vi "Write Curve.vi"(6 "LinkData":T2, 8 "Error In":errorcluster, 9 "Characteristic Curve Values":dbl[](array[numeric]), 10 "Link":T3, 11 "WorkspaceManager":T1) -> (0 "Error Out":errorcluster, 3 "WorkspaceManager out":T1)   [LabVIEW 2011]
uses:
  Controls/ECUMC Item.ctl
  Controls/LinkData.ctl
  <vilib>/NI Veristand/Execution/Workspace/WorkspaceAPI.ctl
  NationalInstruments.VeriStand.ClientAPI
  <vilib>/ECUMC/NIVS/Support Files.llb/Set Char Data (1d, TCP).vi
  <vilib>/NI Veristand/Execution/Workspace/NI VeriStand - Set Multiple Channel Values.vi
  <vilib>/NI Veristand/Execution/Workspace/NI_VS Workspace ExecutionAPI.lvlib
  <vilib>/ECUMC/NIVS/XCPCCP Add-On Execution API.lvlib
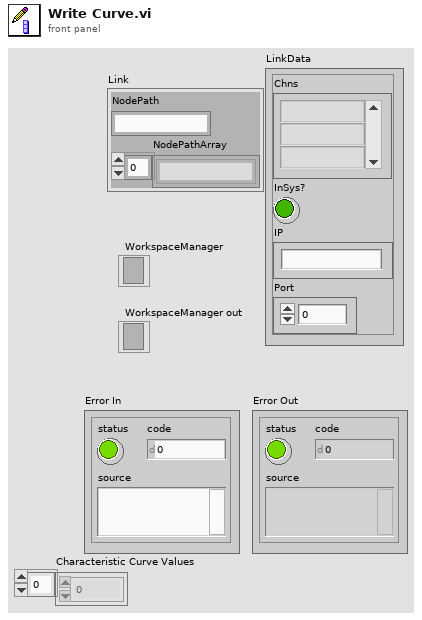
[diagram p1: front panel]
types:
  T1 = typedef "NI_VS Workspace ExecutionAPI.lvlib/WorkspaceAPI.ctl" = refnum<k24>
  T2 = typedef "LinkData.ctl" = cluster{"Chns":string[], "InSys?":bool, "IP":string, "Port":u16}
  T3 = typedef "ECUMC Item.ctl" = cluster{"NodePath":string, "NodePathArray":string[]}
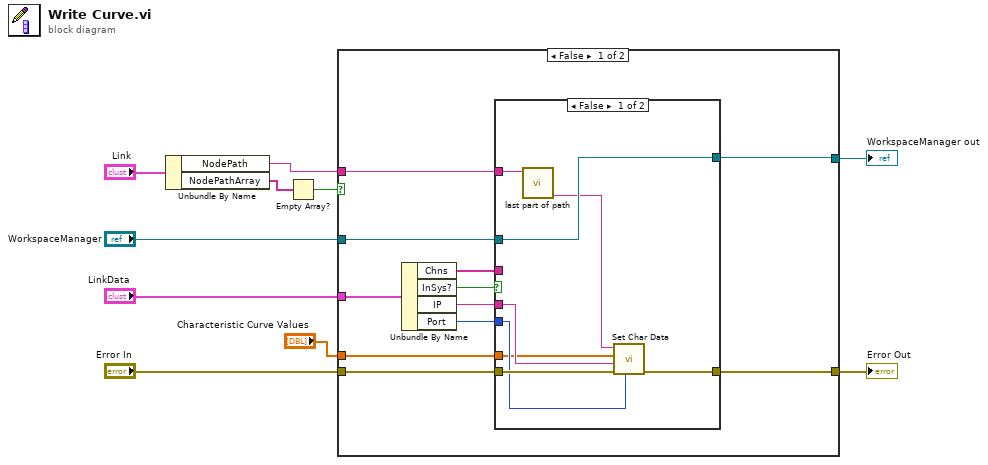
[diagram p0: block diagram]
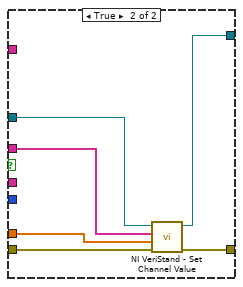
[diagram p2: hidden frame]
diagram:
  n1 = Unbundle By Name("Link") -> ("NodePath"=w7:string, "NodePathArray"=w4:string[])
  n2 = Empty Array?(array=w4) -> (empty?=w3:bool)
  n3 = case shown="False" w3 {
    tunnel: "LinkData" -> [w21 _]
    tunnel: "Error In" -> [w18 w37]
    tunnel: w7 -> [w11 _]
    tunnel: "WorkspaceManager" -> [w15 w36]
    tunnel: [w14 w37] -> w5
    tunnel: [w13 w36] -> w2
    tunnel: "Characteristic Curve Values" -> [w12 _]
    frame False {
      n4 = Unbundle By Name(w21) -> ("Chns"=w19:string[], "InSys?"=w20:bool, "IP"=w17:string, "Port"=w16:u16)
      n5 = case shown="False" w20 {
        tunnel: w19 -> [_ w31]
        tunnel: w15 -> [w25 w35]
        tunnel: w18 -> [w29 w34]
        tunnel: [w28 w33] -> w14
        tunnel: w17 -> [w27 _]
        tunnel: w16 -> [w26 _]
        tunnel: [w25 w32] -> w13
        tunnel: w12 -> [w24 w30]
        tunnel: w11 -> [w23 _]
        frame False {
          n6 = call "last part of path.vi"("String"=w23) -> ("Last Part"=w22:string)  [unwired: 10 in]
          n7 = call-poly <vilib>:"Set Char Data.vi"("Port"=w26, "error in (no error)"=w29, "IP or DNS Name"=w27, "Characteristic Curve Values"=w24, "Characteristic"=w22) -> ("error out"=w28:errorcluster)  [unwired: 6 in]
        }
        frame True {
          n8 = call-poly <vilib>:"NI VeriStand - Set Channel Value.vi"("error in (no error)"=w34, "Values"=w30, "Channels"=w31, "WorkspaceManager in"=w35) -> ("error out"=w33:errorcluster, "WorkspaceManager out"=w32:T1)  [unwired: 6 in]
        }
      }
    }
    frame True {
    }
  }
  "Error Out" <- w5
  "WorkspaceManager out" <- w2
